vi "Save_Info.vi"(8 "error in (no error)":errorcluster, 11 "AB_PackedLibrary in":refnum<class "AB_PackedLibrary.lvclass">) -> (0 "error out":errorcluster, 3 "AB_PackedLibrary out":refnum<class "AB_PackedLibrary.lvclass">)   [LabVIEW 2020, in "AB_PackedLibrary.lvclass"]
uses:
  <vilib>/AppBuilder/AB_Classes/PackedLib/AB_PackedLibrary.lvclass
  e:/builds/penguin/labview/branches/2020/dev/dist/vi.lib/AppBuilder/AB_Classes/Build/AB_Build.lvclass
  <vilib>/AppBuilder/RW_Project/AB_RW_Project_Packed_Lib_Data.ctl
  <vilib>/AppBuilder/RW_Project/AB_RW_Project_PropBag_Action.ctl
  <vilib>/AppBuilder/AB_Classes/PackedLib/AB_PackedLibrary.lvclass/AB_PackedLibrary.ctl
  <vilib>/AppBuilder/AB_Classes/TargetFile/AB_Targetfile.lvclass
  <vilib>/AppBuilder/AB_Classes/Build/AB_Build.lvclass
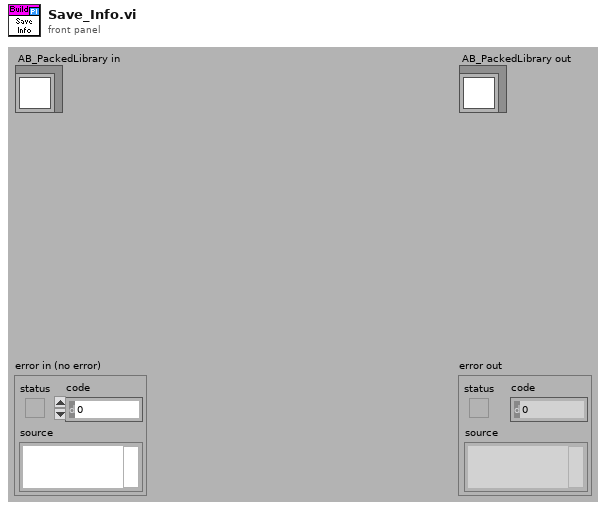
[diagram p1: front panel]
types:
  T1 = typedef "AB_RW_Project_Packed_Lib_Data.ctl" = cluster{"callersAdapt":bool, "showWarnings":bool, "verifyConnpane":bool}
  T2 = typedef "AB_RW_Project_PropBag_Action.ctl" = enum16{"read", "write", "clear", "readPrevious", "writePrevious", "clearPrevious"}
  T3 = typedef "AB_PackedLibrary.ctl" = cluster{"callersAdapt":bool, "showWarnings":bool, "verifyConnpane":bool, "eng_sourceLibrary":string, "eng_packedLib_inMemory":bool}
  T4 = typedef "AB_Build.ctl" = cluster{"buildSpecName":string, "buildSpecDescription":string, "destinations":refnum<class "AB_Destination.lvclass">[], "exclusionOption":T5, "defaultLanguage":string, "supportedLanguages":string[], "excludedDirectories":path[], "buildContext":refnum<vi>, "buildObject":T6, "preview":bool, "programatic":bool, "progressBarEvents":T7, "userLog_Path":path, "preActionID":string, "preAction_Path":path, "postActionID":string, "postAction_Path":path, "eng_checkForBrokenVIs?":bool, "eng_verboseLinkerErrors?":bool, "localDest_Path":path, "targetDest_Path":path, "removeVIObject":u16, "cache":refnum<class "PreviewCache.lvclass">, "use cache":bool, "previewCache_ID":string, "buildCache_ID":string, "eng_TempLocalDest_Path":path, "eng_collectDependencies?":bool, "versionInfo":cluster{"buildVersion":cluster{"major":u16, "minor":u16, "patch":u16, "build":u16}, "autoIncrement":bool}, "eng_enableVIChecksums":bool}
  T5 = typedef "AB_Exclusion_Option.ctl" = cluster{"typedefs":bool, "polymorphicVIs":bool, "unusedLibraryItems":bool, "modifyLibraryFile":bool, "edit-timeDependencies":bool, "inlineVIs":bool, "dependent PPLs":bool, "dependent DLLs":bool}
  T6 = typedef "ItemRef.ctl" = u64
  T7 = typedef "provcom_ProgressBar_Events.ctl" = cluster{"newJob":refnum<user-event>, "newItem":refnum<user-event>, "errorMsg":T8, "cancel":refnum<user-event>}
  T8 = typedef "mxLvBuildError.ctl" = refnum<user-event>
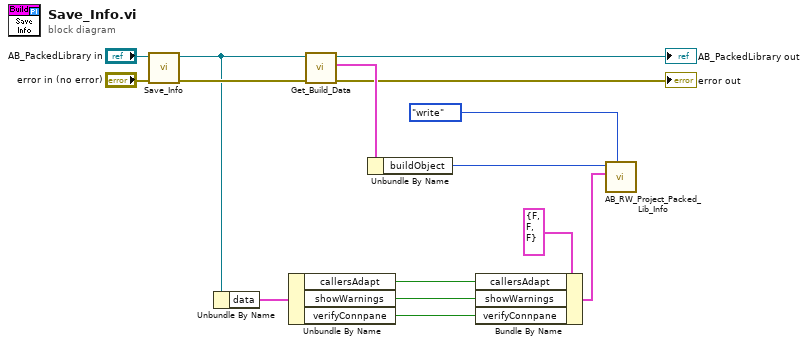
[diagram p0: block diagram]
diagram:
  n1 = call-parent "Save_Info.vi"("error in (no error)"="error in (no error)", "AB_Targetfile in"="AB_PackedLibrary in") -> ("error out"=w11:errorcluster, "AB_Targetfile out"=w10:refnum<class "AB_PackedLibrary.lvclass">)  [unwired: 8 in]
  n2 = Unbundle By Name(w10) -> ("data"=w5:T3)
  n3 = Unbundle By Name(w5) -> ("callersAdapt"=w4:bool, "showWarnings"=w3:bool, "verifyConnpane"=w2:bool)
  n4 = call <vilib>:"Get_Build_Data.vi"("error in (no error)"=w11, "Class in"=w10) -> ("error out"=→"error out":errorcluster, "data"=w13:T4, "Class out"=→"AB_PackedLibrary out":refnum<class "AB_PackedLibrary.lvclass">)  [unwired: 7 in]
  n5 = Unbundle By Name(w13) -> ("buildObject"=w1:T6)
  n6 = Bundle By Name(cluster=T1 {"callersAdapt"=FALSE, "showWarnings"=FALSE, "verifyConnpane"=FALSE} ("PackedLib_info in"), "callersAdapt"=w4, "showWarnings"=w3, "verifyConnpane"=w2) -> (w6:T1)
  n7 = call <vilib>:"AB_RW_Project_Packed_Lib_Info.vi"("action"=AB_RW_Project_PropBag_Action."write", "PackedLib_info in"=w6, "Object In"=w1) -> ()  [unwired: 6 in, 3 out]
